vi "cb_mouseMv.vi"(4 "ctrl_ref":refnum<vi>[](array[refnum]), 5 "이벤트 데이터":cluster{"sender":refnum<k24>, "e":refnum<k24>}, 6 "컨트롤 참조":refnum<k24>, 7 "이벤트 일반 데이터":cluster{"이벤트 소스":i32, "이벤트 타입":u32, "타임스탬프":u32}) -> ()   [LabVIEW 2019]
uses:
  C:/Users/WEGO/Documents/GitHub/Patrolrobot/Subvi/Gmap/dll/GMap.NET.WindowsForms.dll
  Patrolrobot/Subvi/Gmap/dll/GMap.NET.WindowsForms.dll
  System.Windows.Forms
  C:/Users/WEGO/Documents/GitHub/Patrolrobot/Subvi/Gmap/dll/GMap.NET.Core.dll
  Patrolrobot/Subvi/Gmap/dll/GMap.NET.Core.dll
  Ctrl/cmd_common.ctl
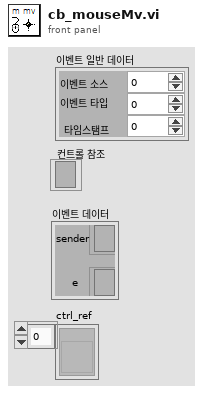
[diagram p1: front panel]
types:
  T1 = typedef "cmd_common.ctl" = enum16{"read", "write"}
  T2 = cluster{"MouseLat":refnum<vi>, "MouseLog":refnum<vi>, "MouseLat_DbClk":refnum<vi>, "MouseLog_DbClk":refnum<vi>, "zoom":refnum<vi>, "PinDropMrkr":refnum<vi>}
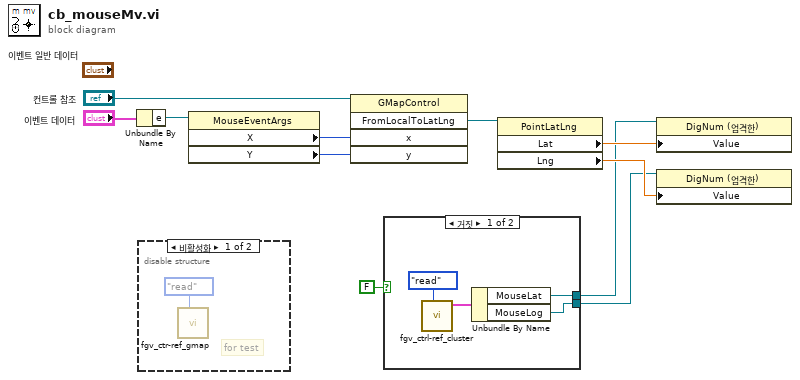
[diagram p0: block diagram]
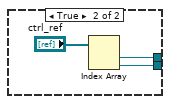
[diagram p3: hidden frame]
diagram:
  n1 = Unbundle By Name("이벤트 데이터") -> ("e"=w6:refnum<k24>)
  n2 = disable-structure shown="비활성화" {
    frame Disabled {
      # "for test"
      n3 = call "fgv_ctr-ref_gmap.vi"("cmd"=cmd_common."read") -> ()  [unwired: 10 in, 1 out]
    }
    frame Enabled {
    }
  }
  n4 = property class="MouseEventArgs"(reference=w6) -> ("X"=w11:i32, "Y"=w10:i32)  [unwired: 1 in, 2 out]
  n5 = invoke class="GMapControl" method="FromLocalToLatLng"(reference="컨트롤 참조", "x"=w11, "y"=w10) -> ("FromLocalToLatLng"=w5:refnum<k24>)  [unwired: 2 in, 4 out]
  n6 = case shown="거짓" FALSE {
    tunnel: [w15 w18] -> w4
    tunnel: [w16 w17] -> w3
    frame False {
      n7 = call "fgv_ctrl-ref_cluster.vi"("cmd"=enum16{"read", "write"}."read") -> ("ref out"=w13:T2)  [unwired: 10 in]
      n8 = Unbundle By Name(w13) -> ("MouseLat"=w16:refnum<vi>, "MouseLog"=w15:refnum<vi>)
    }
    frame True {
      n9 = Index Array(array="ctrl_ref") -> (element #1=w17:refnum<vi>, element #2=w18:refnum<vi>)  [unwired: 2 in]
    }
  }
  n10 = property class="PointLatLng"(reference=w5) -> ("Lat"=w9:dbl, "Lng"=w8:dbl)  [unwired: 1 in, 2 out]
  n11 = property class="DigNum (엄격한)"(reference=w3, "Value"=w9) -> ()  [unwired: 1 in, 2 out]
  n12 = property class="DigNum (엄격한)"(reference=w4, "Value"=w8) -> ()  [unwired: 1 in, 2 out]
